vi "LaserToCSV_v2.vi"() -> ()   [LabVIEW 2016]
uses:
  <instrlib>/Keyence LK-G3000/Public/clusters/LKIF_FLOATVALUE.ctl
  <instrlib>/Keyence LK-G3000/Public/enums/LKIF_FLOATRESULT.ctl
  <vilib>/Utility/file.llb/Write Delimited Spreadsheet (DBL).vi
  <instrlib>/Keyence LK-G3000/Keyence LK-G3000.lvlib
panel:
  in  "Timing":u32=100
  out "CalcData2":T1 {"LKIF_FLOATRESULT" items=["VALID", "RANGEOVER_P", "RANGEOVER_N", "WAITING"]}
  out "CalcData1":T1 {"LKIF_FLOATRESULT" items=["VALID", "RANGEOVER_P", "RANGEOVER_N", "WAITING"]}
  out "Trend Graph":cluster{"Value":sgl, "Value":sgl}(graph)
  in  "Stop VI":bool
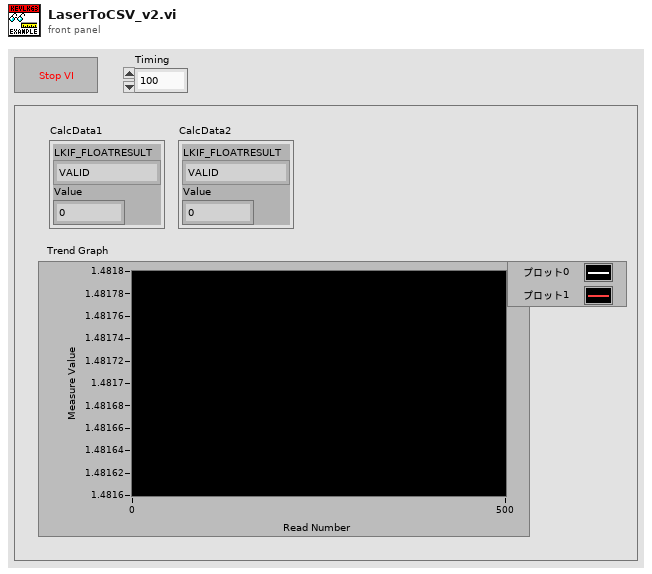
[diagram p1: front panel]
types:
  T1 = typedef "Keyence LK-G3000.lvlib/LKIF_FLOATVALUE.ctl" = cluster{"LKIF_FLOATRESULT":T2, "Value":sgl}
  T2 = typedef "Keyence LK-G3000.lvlib/LKIF_FLOATRESULT.ctl" = i32
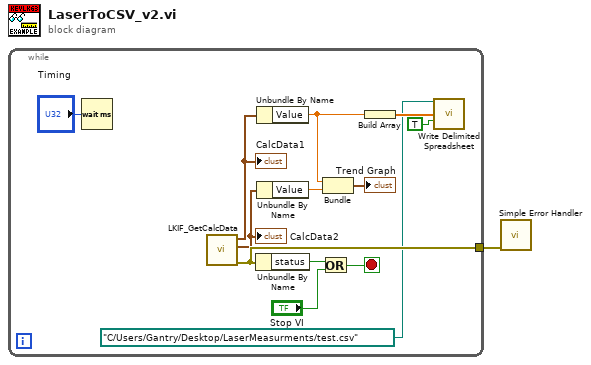
[diagram p0: block diagram]
diagram:
  n1 = while {
    tunnel: [w13] -> w1
    stop <- w14 stop-if-true
    n2 = Wait (ms)(milliseconds to wait="Timing") -> ()  [unwired: 1 out]
    n3 = call <instrlib>:"LKIF_GetCalcData.vi"() -> ("error out"=w13:errorcluster, "CalcData2"=w9:T1, "CalcData1"=w10:T1)  [unwired: 9 in]
    "CalcData1" <- w10
    "CalcData2" <- w9
    n4 = Unbundle By Name(w13) -> ("status"=w12:bool)
    n5 = Unbundle By Name(w10) -> ("Value"=w6:sgl)
    n6 = Unbundle By Name(w9) -> ("Value"=w8:sgl)
    n7 = Or(x=w12, y="Stop VI") -> (x .or. y?=w14:bool)
    n8 = Bundle("Value"=w6, "Value"=w8) -> (→"Trend Graph":cluster{"Value":sgl, "Value":sgl})  [unwired: 1 in]
    n9 = Build Array(w6) -> (w5:sgl[])
    n10 = call-poly <vilib>:"Write Delimited Spreadsheet.vi"("file path (dialog if empty)"=path "C:/Users/Gantry/Desktop/LaserMeasurments/test.csv", "1D data"=w5, "append to file? (new file:F)"=TRUE) -> ()  [unwired: 11 in, 2 out]
  }
  n11 = call <vilib>:"Simple Error Handler.vi"("error in (no error)"=w1) -> ()  [unwired: 4 in, 5 out]
